vi "generateimagejmacro.vi"(7 "file format":T1, 11 "T:galvo F:resonant default:T":bool=TRUE) -> ()   [LabVIEW 2012]
uses:
  Custom Controls/file format type def.ctl
  GFG/GFGpathGet.vi
  GFG/GFGnumericGet.vi
  GFG/GFGbooleanGet.vi
  GFG/GFG library.lvlib
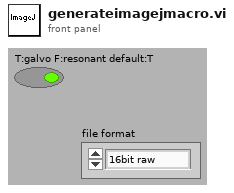
[diagram p1: front panel]
types:
  T1 = typedef "file format type def.ctl" = enum16{"16bit raw", "32bit raw", "16bit multi-tiff (interleave)", "16bit multi-tiff (separate)", "16bit multi-tiff (stacked)", "32bit multi-tiff (interleave)", "32bit multi-tiff (separate)", "32bit multi-tiff (stacked)", "16bit tiff series (interleave)", "16bit tiff series (separate)", "16bit tiff series (stacked)", "32bit tiff series (interleave)", "32bit tiff series (separate)", "32bit tiff series (stacked)"}
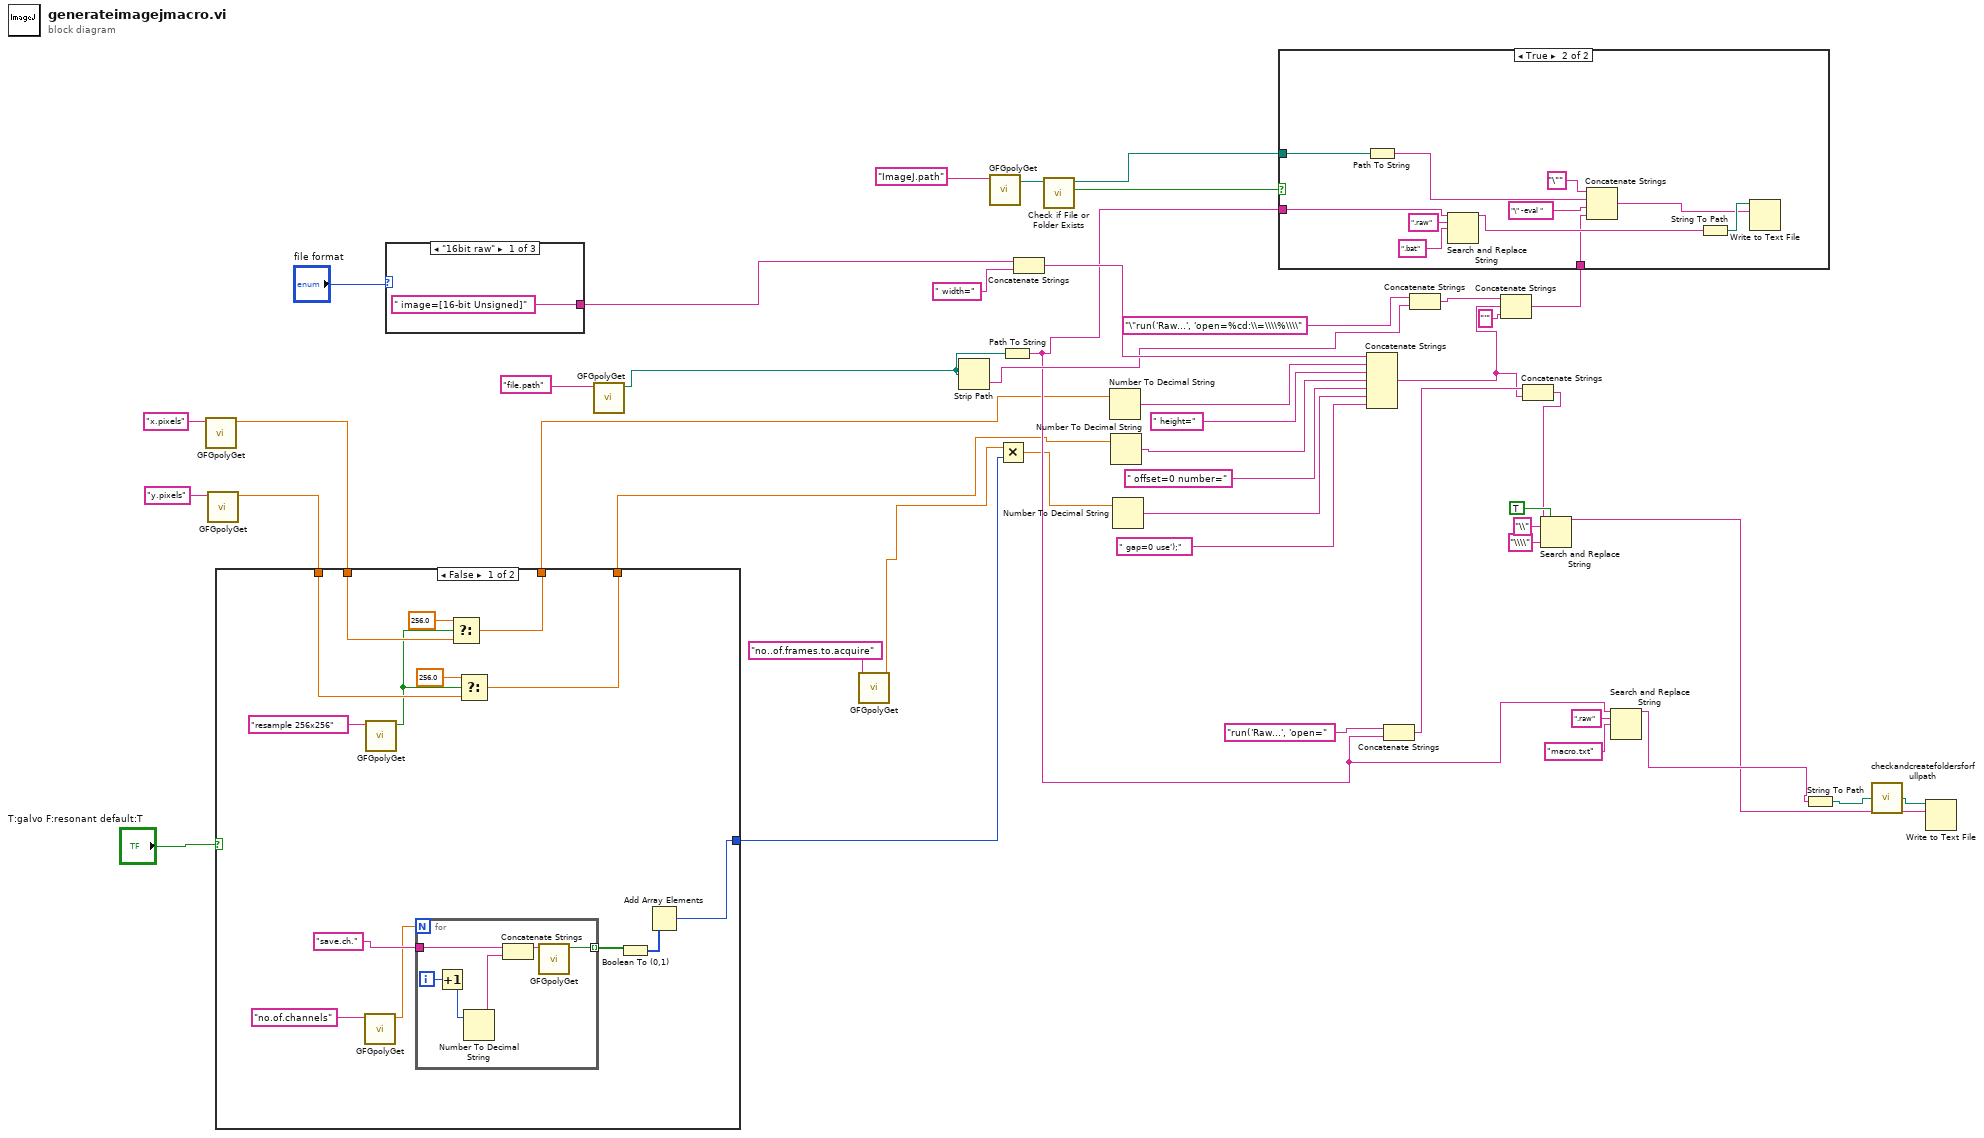
[diagram p0: block diagram]
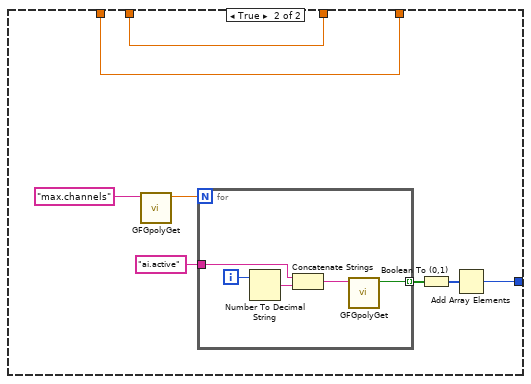
[diagram p2: hidden frame]
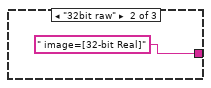
[diagram p4: hidden frame]
diagram:
  n1 = call-poly "GFGpolyGet.vi"("Variable Name in"="x.pixels") -> ("Numeric"=w2:dbl)  [unwired: 9 in, 1 out]
  n2 = call-poly "GFGpolyGet.vi"("Variable Name in"="y.pixels") -> ("Numeric"=w4:dbl)  [unwired: 9 in, 1 out]
  n3 = case shown="False" "T:galvo F:resonant default:T" {
    tunnel: [w49 w69] -> w15
    tunnel: [w53 w68] -> w3
    tunnel: w4 -> [w55 w68]
    tunnel: [w56 w67] -> w1
    tunnel: w2 -> [w57 w67]
    frame False {
      n4 = call-poly "GFGpolyGet.vi"("Variable Name in"="no.of.channels" ("Tag in")) -> ("Numeric"=w47:dbl)  [unwired: 9 in, 1 out]
      n5 = call-poly "GFGpolyGet.vi"("Variable Name in"="resample 256x256") -> ("Boolean"=w54:bool)  [unwired: 10 in]
      n6 = for {
        N: w47 -> [_]
        tunnel: "save.ch." ("Variable Name in") -> [w66]
        tunnel: [w65] -> w51 mode=indexing
        i -> [w64]
        n7 = Increment(x=w64) -> (x+1=w63:i32)
        n8 = Number To Decimal String(number=w63) -> (decimal integer string=w61:string)  [unwired: 1 in]
        n9 = Concatenate Strings(w66, w61) -> (w62:string)
        n10 = call-poly "GFGpolyGet.vi"("Variable Name in"=w62) -> ("Boolean"=w65:bool)  [unwired: 10 in]
      }
      n11 = Select(t=256.0, s=w54, f=w57) -> (s? t:f=w56:dbl)
      n12 = Select(t=256.0, s=w54, f=w55) -> (s? t:f=w53:dbl)
      n13 = Boolean To (0,1)(Boolean=w51) -> (0, 1=w50:i16[])
      n14 = Add Array Elements(numeric array=w50) -> (sum=w49:i16)
    }
    frame True {
      n15 = call-poly "GFGpolyGet.vi"("Variable Name in"="max.channels") -> ("Numeric"=w73:dbl)  [unwired: 9 in, 1 out]
      n16 = for {
        N: w73 -> [_]
        tunnel: [w79] -> w71 mode=indexing
        tunnel: "ai.active" ("Variable Name in") -> [w78]
        i -> [w77]
        n17 = Number To Decimal String(number=w77) -> (decimal integer string=w76:string)  [unwired: 1 in]
        n18 = Concatenate Strings(w78, w76) -> (w75:string)
        n19 = call-poly "GFGpolyGet.vi"("Variable Name in"=w75) -> ("Boolean"=w79:bool)  [unwired: 10 in]
      }
      n20 = Boolean To (0,1)(Boolean=w71) -> (0, 1=w70:i16[])
      n21 = Add Array Elements(numeric array=w70) -> (sum=w69:i16)
    }
  }
  n22 = case shown="\"16bit raw\"" "file format" {
    tunnel: [" image=[16-bit Unsigned]" ("image type") " image=[32-bit Real]" ("image type") _] -> w18
    frame "16bit raw" {
    }
    frame "32bit raw" {
    }
    frame Default {
    }
  }
  n23 = call-poly "GFGpolyGet.vi"("Variable Name in"="file.path" ("Tag in")) -> ("Path"=w20:path)  [unwired: 9 in, 1 out]
  n24 = call-poly "GFGpolyGet.vi"("Variable Name in"="no..of.frames.to.acquire") -> ("Numeric"=w7:dbl)  [unwired: 9 in, 1 out]
  n25 = Strip Path(path=w20) -> (name=w37:string)  [unwired: 1 out]
  n26 = call-poly "GFGpolyGet.vi"("Variable Name in"="ImageJ.path" ("Tag in")) -> ("Path"=w13:path)  [unwired: 9 in, 1 out]
  n27 = Multiply(x=w7, y=w15) -> (x*y=w6:dbl)
  n28 = Path To String(path=w20) -> (string=w28:string)
  n29 = Concatenate Strings(w18, " width=" ("string")) -> (w39:string)
  n30 = call <vilib>:"Check if File or Folder Exists.vi"("path"=w13) -> ("file or folder exists?"=w12:bool, "dup path"=w11:path)  [unwired: 8 in, 1 out]
  n31 = Number To Decimal String(number=w1) -> (decimal integer string=w46:string)  [unwired: 1 in]
  n32 = Number To Decimal String(number=w3) -> (decimal integer string=w44:string)  [unwired: 1 in]
  n33 = Number To Decimal String(number=w6) -> (decimal integer string=w42:string)  [unwired: 1 in]
  n34 = Concatenate Strings(w39, w46, " height=", w44, " offset=0 number=", w42, " gap=0 use');") -> (w31:string)
  n35 = Concatenate Strings("run('Raw...', 'open=", w28) -> (w32:string)
  n36 = Concatenate Strings("\"run('Raw...', 'open=%cd:\\=\\\\%\\\\", w37) -> (w36:string)
  n37 = Concatenate Strings(w36, w31, "'" ("string")) -> (w34:string)
  n38 = case shown="True" w12 {
    tunnel: w34 -> [_ w86]
    tunnel: w28 -> [_ w85]
    tunnel: w11 -> [_ w84]
    frame False {
    }
    frame True {
      n39 = Path To String(path=w84) -> (string=w83:string)
      n40 = Search and Replace String(input string=w85, search string=".raw", replace string=".bat" ("string")) -> (result string=w88:string)  [unwired: 5 in, 3 out]
      n41 = Concatenate Strings("\"" ("string"), w83, "\" -eval " ("string"), w86) -> (w87:string)
      n42 = String To Path(string=w88) -> (path=w89:path)
      n43 = Write to Text File(file (use dialog)=w89, text=w87) -> ()  [unwired: 2 in, 3 out]
    }
  }
  n44 = Concatenate Strings(w32, w31) -> (w24:string)
  n45 = Search and Replace String(replace all?=TRUE ("replace all? (F)"), input string=w24, search string="\\", replace string="\\\\" ("replace string (\"\")")) -> (result string=w22:string)  [unwired: 4 in, 3 out]
  n46 = Search and Replace String(input string=w28, search string=".raw", replace string="macro.txt" ("string")) -> (result string=w23:string)  [unwired: 5 in, 3 out]
  n47 = String To Path(string=w23) -> (path=w9:path)
  n48 = call "checkandcreatefoldersforfullpath.vi"("Path IN"=w9) -> ("Path OUT"=w8:path)  [unwired: 4 in]
  n49 = Write to Text File(file (use dialog)=w8, text=w22) -> ()  [unwired: 2 in, 3 out]
